vi "Measurement.PhotocurrentMapping.GetConfiguration.vi"(8 "error in (no error)":errorcluster, 11 "Measurement.PhotocurrentMapping":refnum<class "Measurement.PhotocurrentMapping.lvclass">) -> (0 "error out":errorcluster, 2 "Configuration":T1={"Measurement.Type"=enum."Free", "Hardware"={"SMU"={"Enable"=FALSE, "SMU Model"="", "Configuration"={"VISA Resource"="", "Channel"=""}}, "LIA"={"Enable"=FALSE, "LIA Model"="", "Configuration"={"VISA Resource"=""}}, "XYStage"={"Enable"=FALSE, "XYStage Model"="", "Configuration"={"Serial Number"="", "X Axis"="", "Y Axis"="", "Real-World Units"="", "Counts per Unit"=1}}}, "Measurement"={"X"={"Start, units"=-10000.0, "Stop, units"=10000.0, "Step, units"=250.0}, "Y"={"Start, units"=-10000.0, "Stop, units"=10000.0, "Step, units"=250.0}, "Accumulation"=5}} {"Measurement"."Accumulation" step=1; "Measurement"."Y"."Step, units" step=100.0 format="%#_6f"; "Measurement"."Y"."Stop, units" step=100.0 format="%#_6f"; "Measurement"."Y"."Start, units" step=100.0 format="%#_6f"; "Measurement"."X"."Step, units" step=100.0 format="%#_6f"; "Measurement"."X"."Stop, units" step=100.0 format="%#_6f"; "Measurement"."X"."Start, units" step=100.0 format="%#_6f"}, 3 "Measurement.PhotocurrentMapping out":refnum<class "Measurement.PhotocurrentMapping.lvclass">)   [LabVIEW 2017, in "Measurement.PhotocurrentMapping.lvclass"]
doc: "---------------------------------------------------------------\nJKI State Machine Objects™\nhttp://jki.net/state-machine-objects/\nCopyright (C) 2005-2015, JKI <info@jki.net>\nALL RIGHTS RESERVEDJKI State Machine Objects (SMO) 1.0.0.5\nJKI - JKI\nCopyright (c) 2016, JKI"
uses:
  Measurement.PhotocurrentMapping.lvclass
  Typedefs/Configuration--Cluster.ctl
  Measurement/Typedefs/Measurement.Type--Enum.ctl
  Typedefs/Configuration.Hardware--Cluster.ctl
  Measurement/Typedefs/Configuration.SMU--Cluster.ctl
  SMU/Typedefs/Configuration--Cluster.ctl
  Measurement/Typedefs/Configuration.LIA--Cluster.ctl
  LIA/Typedefs/Configuration--Cluster.ctl
  Measurement/Typedefs/Configuration.XYStage--Cluster.ctl
  XYStage/Typedefs/Configuration--Cluster.ctl
  Typedefs/Configuration.Measurement--Cluster.ctl
  Typedefs/Configuration.Axis--Cluster.ctl
  Measurement.PhotocurrentMapping.lvclass/Measurement.PhotocurrentMapping.ctl
  Measurement/Measurement.lvclass
  SMU/SMU.lvclass
  LIA/LIA.lvclass
  XYStage/XYStage.lvclass
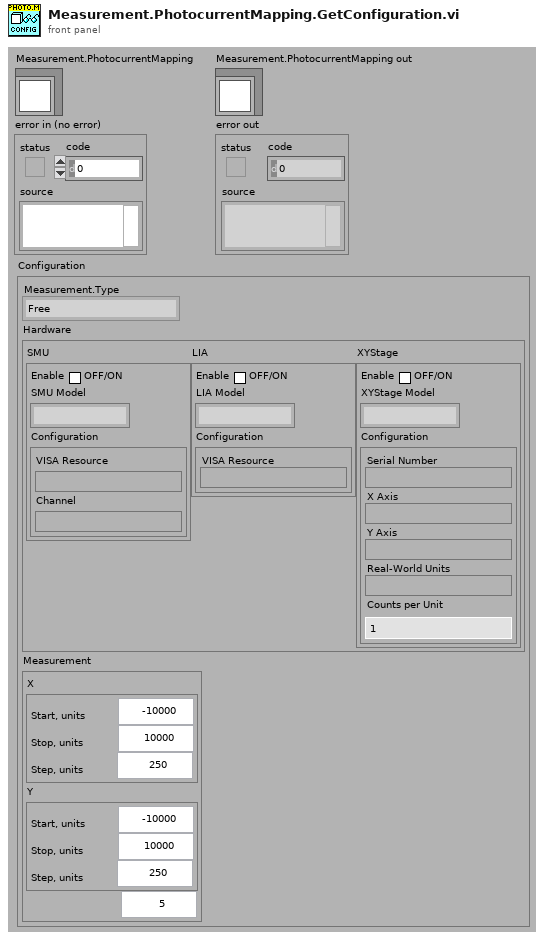
[diagram p1: front panel]
types:
  T1 = typedef "Measurement.PhotocurrentMapping.lvclass/Configuration--Cluster.ctl" = cluster{"Measurement.Type":T2, "Hardware":T3, "Measurement":T10}
  T2 = typedef "Measurement.lvclass/Measurement.Type--Enum.ctl" = enum16{"Free", "I/V Curve", "Wavelength sweeping", "Photocurrent mapping"}
  T3 = typedef "Measurement.PhotocurrentMapping.lvclass/Configuration.Hardware--Cluster.ctl" = cluster{"SMU":T4, "LIA":T6, "XYStage":T8}
  T4 = typedef "Measurement.lvclass/Configuration.SMU--Cluster.ctl" = cluster{"Enable":bool, "SMU Model":string, "Configuration":T5}
  T5 = typedef "SMU.lvclass/Configuration--Cluster.ctl" = cluster{"VISA Resource":string, "Channel":string}
  T6 = typedef "Measurement.lvclass/Configuration.LIA--Cluster.ctl" = cluster{"Enable":bool, "LIA Model":string, "Configuration":T7}
  T7 = typedef "LIA.lvclass/Configuration--Cluster.ctl" = cluster{"VISA Resource":string}
  T8 = typedef "Measurement.lvclass/Configuration.XYStage--Cluster.ctl" = cluster{"Enable":bool, "XYStage Model":string, "Configuration":T9}
  T9 = typedef "XYStage.lvclass/Configuration--Cluster.ctl" = cluster{"Serial Number":string, "X Axis":string, "Y Axis":string, "Real-World Units":string, "Counts per Unit":u32}
  T10 = typedef "Measurement.PhotocurrentMapping.lvclass/Configuration.Measurement--Cluster.ctl" = cluster{"X":T11, "Y":T11, "Accumulation":u16}
  T11 = typedef "Measurement.PhotocurrentMapping.lvclass/Configuration.Axis--Cluster.ctl" = cluster{"Start, units":dbl, "Stop, units":dbl, "Step, units":dbl}
  T12 = typedef "Measurement.PhotocurrentMapping.lvclass/PrivateData--Ref.ctl" = refnum<data-value>
  T13 = typedef "Measurement.PhotocurrentMapping.lvclass/PrivateData--Cluster.ctl" = cluster{"Configuration":T1, "Dependencies":T14}
  T14 = typedef "Measurement.PhotocurrentMapping.lvclass/Dependencies--Cluster.ctl" = cluster{"SMU":refnum<class "SMU.lvclass">, "LIA":refnum<class "LIA.lvclass">, "XYStage":refnum<class "XYStage.lvclass">}
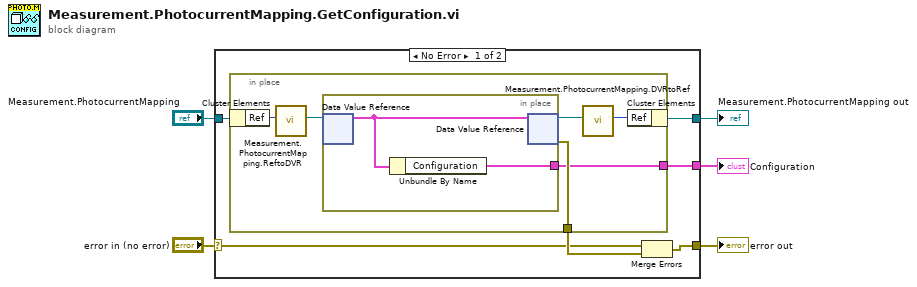
[diagram p0: block diagram]
diagram:
  n1 = case shown="No Error" "error in (no error)" {
    selector: "error in (no error)" -> [w7 w20]
    tunnel: "Measurement.PhotocurrentMapping" -> [w8 w21]
    tunnel: [w9 w20] -> w4
    tunnel: [w11 w21] -> w3
    tunnel: [w6 _] -> w1
    frame No Error {
      n2 = in-place {
        in-place-border: [w17] -> w10
        in-place-border: [w12] -> w6
        n3 = in-place-cluster #1(w8) -> ("Ref"=w16:u32)
        n4 = call "Measurement.PhotocurrentMapping.ReftoDVR.vi"("Ref"=w16) -> ("Ref"=w15:T12)  [unwired: 10 in]
        n5 = in-place {
          in-place-border: [w18] -> w12
          n6 = in-place-dvr #2(w15) -> (w19:T13)  [unwired: 1 out]
          n7 = Unbundle By Name(w19) -> ("Configuration"=w18:T1)
          n8 = in-place-dvr #2(w19) -> (w14:T12, w17:errorcluster)
        }
        n9 = call "Measurement.PhotocurrentMapping.DVRtoRef.vi"("Ref"=w14) -> ("Ref"=w13:u32)  [unwired: 10 in]
        n10 = in-place-cluster #1("Ref"=w13) -> (w11:refnum<class "Measurement.PhotocurrentMapping.lvclass">)
      }
      n11 = Merge Errors(w7, w10) -> (w9:errorcluster)
    }
    frame Error {
    }
  }
  "error out" <- w4
  "Measurement.PhotocurrentMapping out" <- w3
  "Configuration" <- w1
